vi "Remote control Client ver 0.1.vi"() -> ()   [LabVIEW 2018]
panel:
  out "error out":errorcluster
  in  "stop":bool
  out "Image":T1(plugin-control)
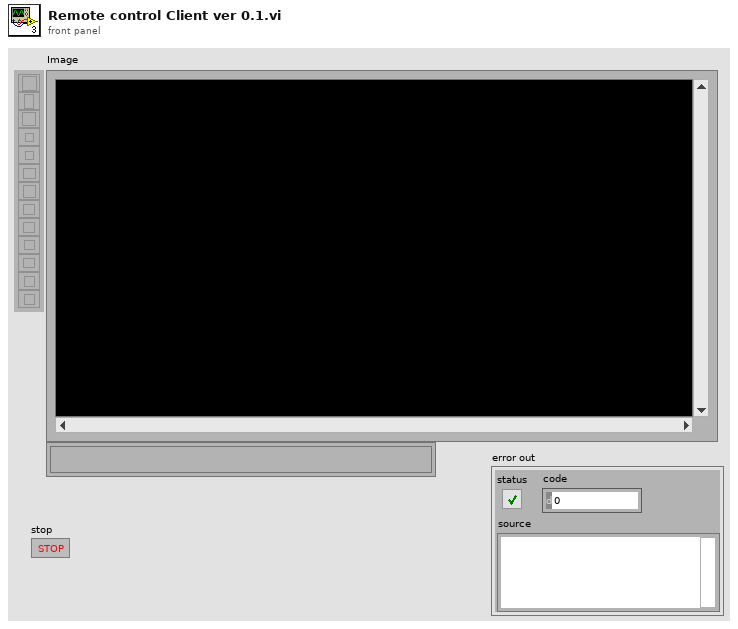
[diagram p1: front panel]
types:
  T1 = typedef "IMAQ Image.ctl" = refnum<image>
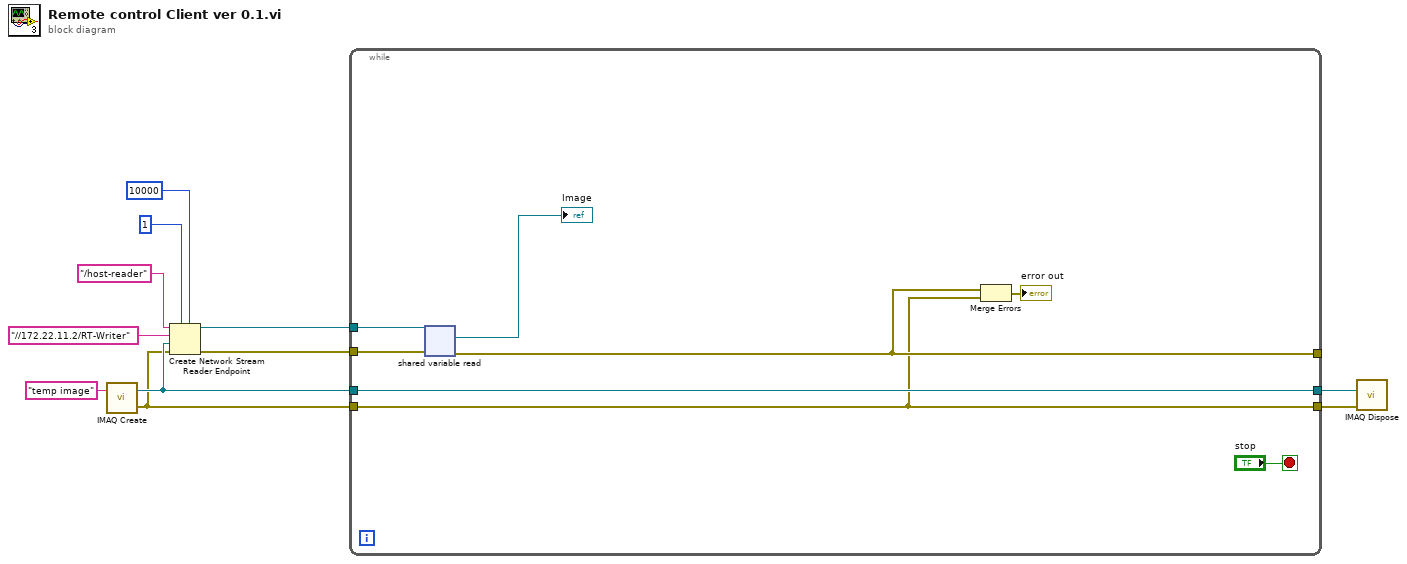
[diagram p0: block diagram]
diagram:
  n1 = call "IMAQ Create"("Image Name"="temp image") -> ("New Image"=w5:T1, "error out"=w2:errorcluster)  [unwired: 4 in]
  n2 = Create Network Stream Reader Endpoint(5:10000 ("timeout in ms (-1)"), 7:1 ("reader buffer size"), 8:w2, 9:w5, 10:"//172.22.11.2/RT-Writer" ("reader name"), 11:"/host-reader" ("writer name")) -> (0:w6:errorcluster, 3:w7:refnum<k21>)  [unwired: 1 in]
  n3 = while {
    tunnel: w7 -> [w19]
    tunnel: w6 -> [w18]
    tunnel: w2 -> [w13]
    tunnel: [w13] -> w3
    tunnel: [w14] -> _
    tunnel: [w15] -> w4
    tunnel: w5 -> [w15]
    stop <- "stop" stop-if-true
    n4 = shared-variable-read(w19, w18) -> (w14:errorcluster, →"Image":T1)  [unwired: 1 in, 2 out]
    n5 = Merge Errors(w14, w13) -> (→"error out":errorcluster)
  }
  n6 = call "IMAQ Dispose"("Image"=w4, "error in (no error)"=w3) -> ()  [unwired: 4 in, 1 out]
